vi "LEDRincController.vi"() -> ()   [LabVIEW 2024]
uses:
  <vilib>/Instr/_visa.llb/VISA Configure Serial Port (Instr).vi
panel:
  in  "stop 2":bool
  in  "stop":bool
  in  "Enum":enum16{"Idle", "Off", "Block", "Access"}(ring)
  in  "Port":refnum<visa-resource-name>
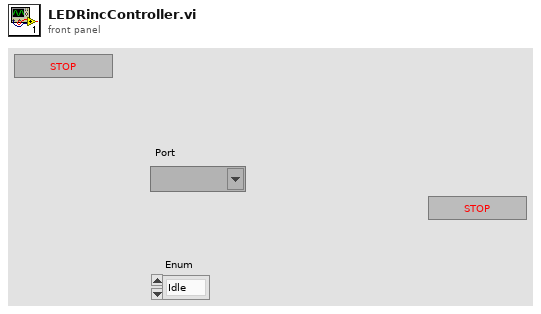
[diagram p1: front panel]
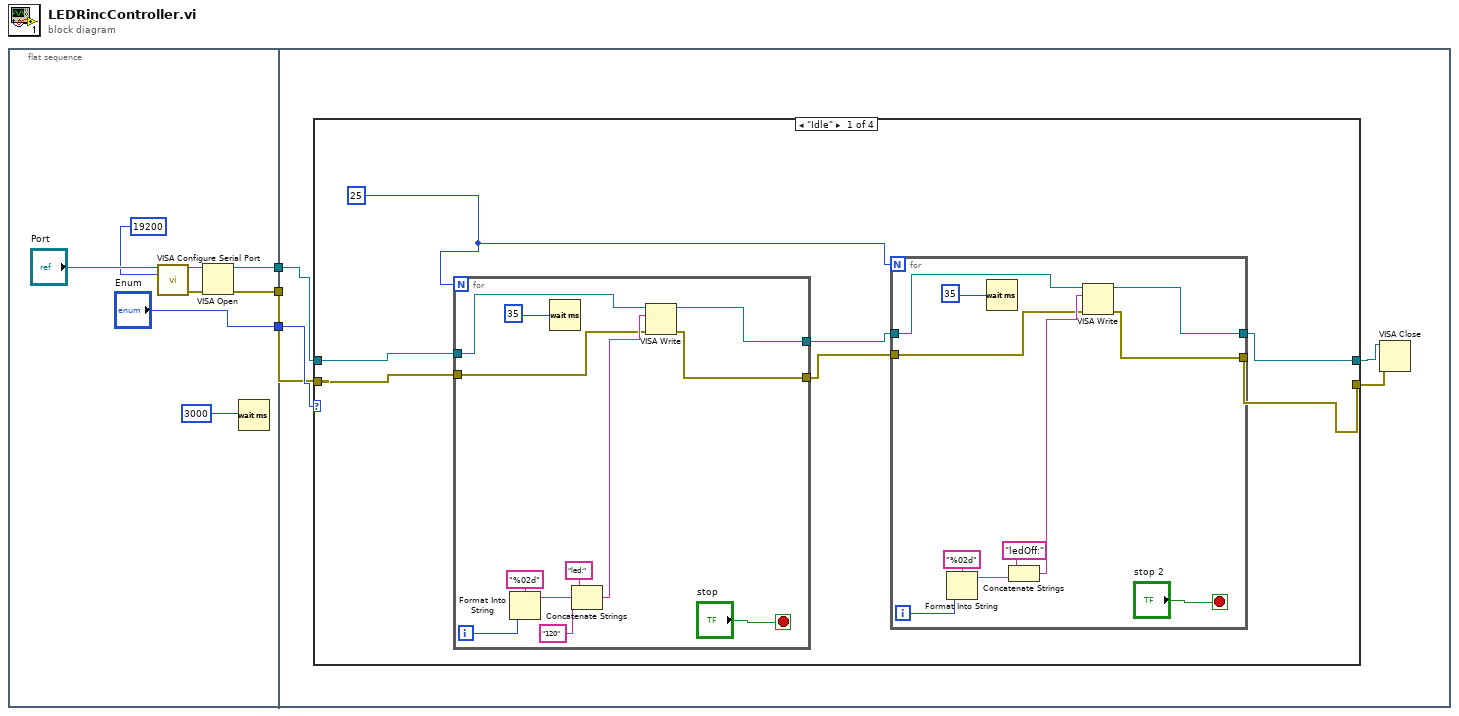
[diagram p0: block diagram]
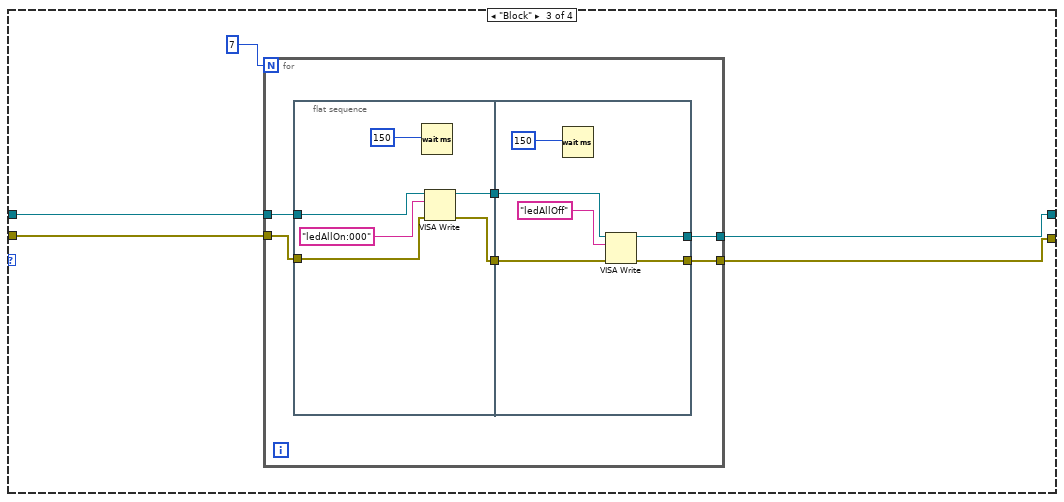
[diagram p3: hidden frame]
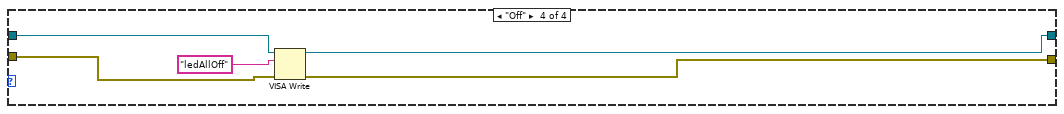
[diagram p4: hidden frame]
diagram:
  n1 = flat-sequence {
    tunnel: ["Enum"] -> w3
    tunnel: [w6] -> w2
    tunnel: [w5] -> w1
    tunnel: w3 -> [w16]
    tunnel: w2 -> [w15]
    tunnel: w1 -> [w14]
    frame #0 {
      n2 = call-poly "VISA Configure Serial Port"("VISA resource name"="Port", "baud rate (9600)"=u32 19200) -> ("VISA resource name out"=w10:refnum<visa-resource-name>, "error out"=w9:errorcluster)  [unwired: 12 in]
      n3 = VISA Open(error in (no error)=w9, VISA resource name=w10) -> (VISA resource name=w6:refnum<visa-resource-name>, error out=w5:errorcluster)  [unwired: 3 in]
      n4 = Wait (ms)(milliseconds to wait=u32 3000 ("millisecond multiple")) -> ()  [unwired: 1 out]
    }
    frame #1 {
      n5 = case shown="\"Idle\"" w16 {
        tunnel: w15 -> [w22 w48 w52 w75]
        tunnel: w14 -> [w23 w47 w51 w74]
        tunnel: [w19 w48 w50 w73] -> w12
        tunnel: [w18 w47 w49 w72] -> w13
        frame "Idle" {
          w17 = 25
          n6 = for {
            N: w17 -> [_]
            tunnel: w23 -> [w37]
            tunnel: w22 -> [w38]
            tunnel: [w40] -> w20
            tunnel: [w41] -> w21
            i -> [w45]
            stop <- "stop" stop-if-true
            n7 = Format Into String(format string="%02d", w45) -> (resulting string=w35:string)  [unwired: 2 in, 1 out]
            n8 = Wait (ms)(milliseconds to wait=u32 35 ("millisecond multiple")) -> ()  [unwired: 1 out]
            n9 = Concatenate Strings("led:", w35, "120") -> (w42:string)
            n10 = VISA Write(VISA resource name=w38, write buffer=w42, error in (no error)=w37) -> (VISA resource name out=w41:refnum<visa-resource-name>, error out=w40:errorcluster)  [unwired: 1 out]
          }
          n11 = for {
            N: w17 -> [_]
            tunnel: w20 -> [w26]
            tunnel: w21 -> [w27]
            tunnel: [w29] -> w18
            tunnel: [w30] -> w19
            i -> [w33]
            stop <- "stop 2" stop-if-true
            n12 = Format Into String(format string="%02d", w33) -> (resulting string=w24:string)  [unwired: 2 in, 1 out]
            n13 = Wait (ms)(milliseconds to wait=u32 35 ("millisecond multiple")) -> ()  [unwired: 1 out]
            n14 = Concatenate Strings("ledOff:", w24) -> (w31:string)
            n15 = VISA Write(VISA resource name=w27, write buffer=w31, error in (no error)=w26) -> (VISA resource name out=w30:refnum<visa-resource-name>, error out=w29:errorcluster)  [unwired: 1 out]
          }
        }
        frame "Access" {
        }
        frame "Block" {
          n16 = for {
            N: 7 -> [_]
            tunnel: w52 -> [w57]
            tunnel: w51 -> [w56]
            tunnel: [w55] -> w50
            tunnel: [w54] -> w49
            n17 = flat-sequence {
              tunnel: [w63] -> w59
              tunnel: [w62] -> w58
              tunnel: w57 -> [w61]
              tunnel: w56 -> [w60]
              tunnel: w59 -> [w70]
              tunnel: w58 -> [w69]
              tunnel: [w68] -> w55
              tunnel: [w67] -> w54
              frame #0 {
                n18 = Wait (ms)(milliseconds to wait=u32 150 ("millisecond multiple")) -> ()  [unwired: 1 out]
                n19 = VISA Write(VISA resource name=w61, write buffer="ledAllOn:000", error in (no error)=w60) -> (VISA resource name out=w63:refnum<visa-resource-name>, error out=w62:errorcluster)  [unwired: 1 out]
              }
              frame #1 {
                n20 = Wait (ms)(milliseconds to wait=u32 150 ("millisecond multiple")) -> ()  [unwired: 1 out]
                n21 = VISA Write(VISA resource name=w70, write buffer="ledAllOff", error in (no error)=w69) -> (VISA resource name out=w68:refnum<visa-resource-name>, error out=w67:errorcluster)  [unwired: 1 out]
              }
            }
          }
        }
        frame "Off" {
          n22 = VISA Write(VISA resource name=w75, write buffer="ledAllOff", error in (no error)=w74) -> (VISA resource name out=w73:refnum<visa-resource-name>, error out=w72:errorcluster)  [unwired: 1 out]
        }
      }
      n23 = VISA Close(VISA resource name=w12, error in (no error)=w13) -> ()  [unwired: 1 out]
    }
  }
